vi "LTA-HS-testing2.vi"() -> ()   [LabVIEW 2013]
uses:
  <vilib>/Utility/error.llb/DialogType.ctl
panel:
  out "Current position":dbl
  out "error IO 2":errorcluster
  out "Motion Time (s)":dbl
  in  "Position":dbl
  in  "error IO":errorcluster
  in  "VISA resource name":refnum<visa-resource-name>
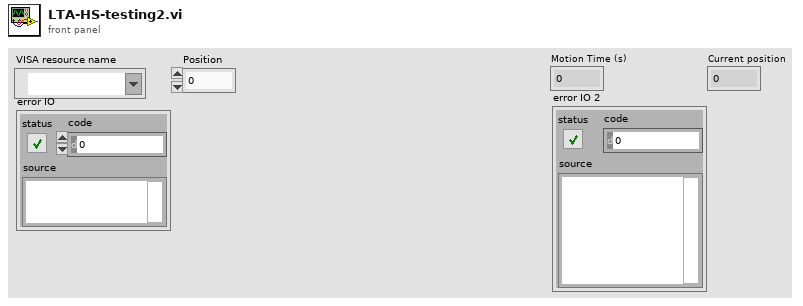
[diagram p1: front panel]
types:
  T1 = cluster{"VISA resource name":refnum<visa-resource-name>, string, i32, "error out":errorcluster}
  T2 = cluster{"VISA resource name":refnum<visa-resource-name>, "Device name":string, "Controller address":i32, "error":errorcluster}
  T3 = typedef "DialogType.ctl" = u16
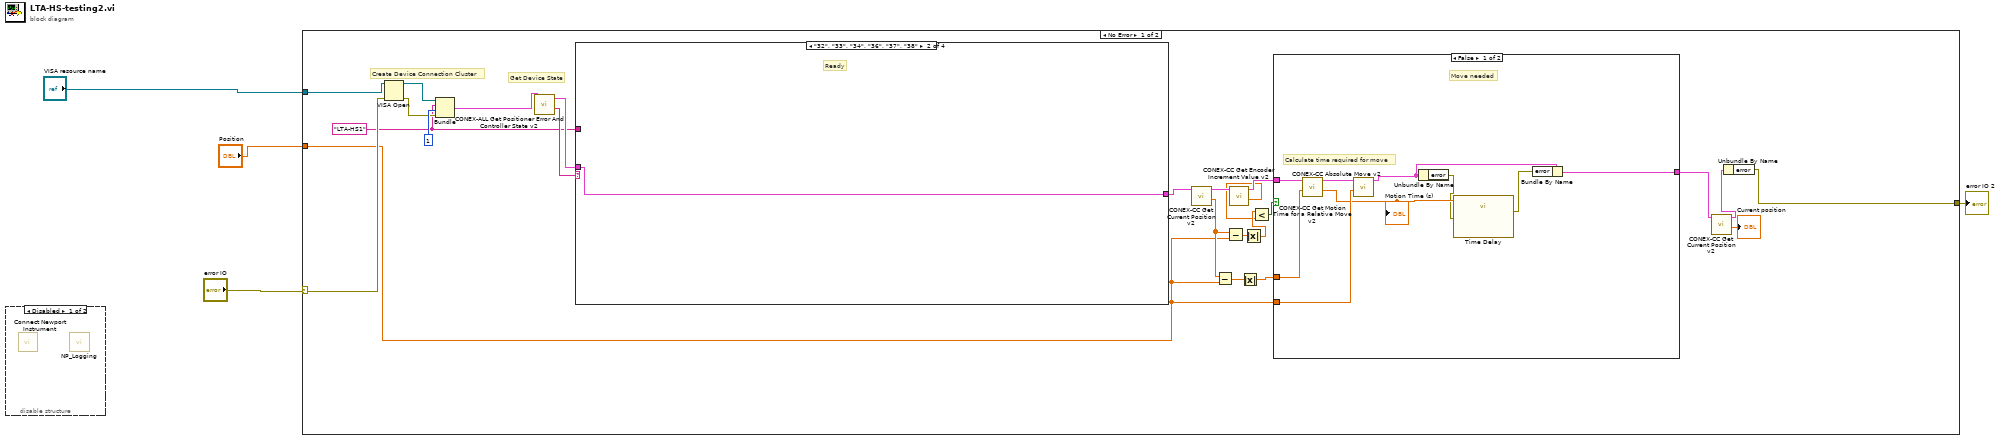
[diagram p0: block diagram]
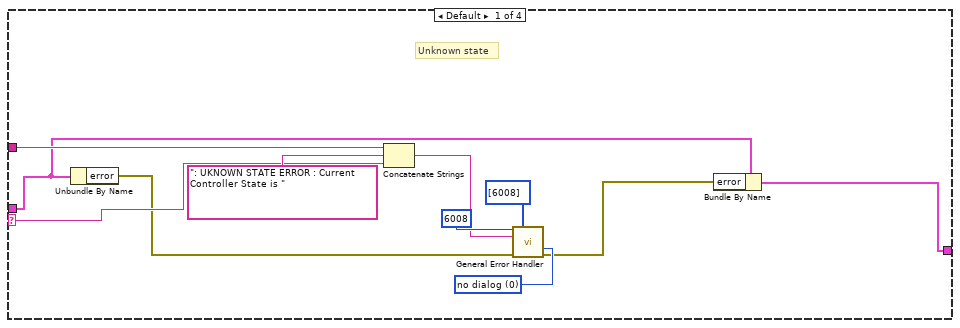
[diagram p4: hidden frame]
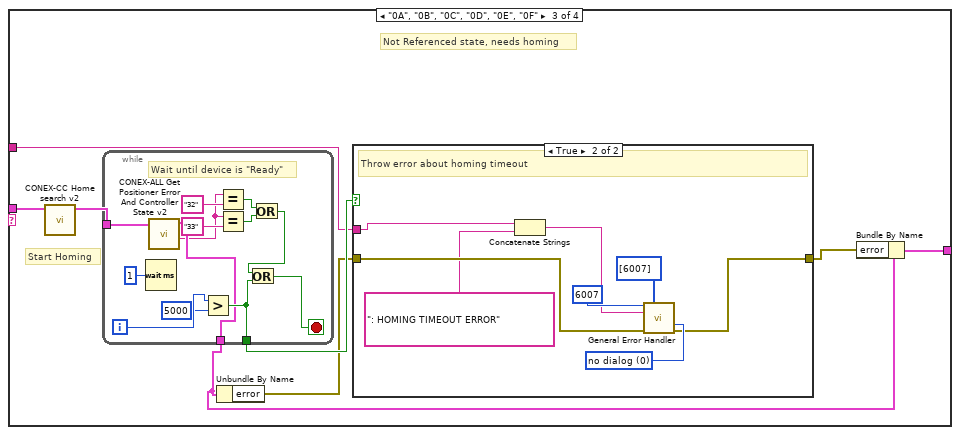
[diagram p5: hidden frame]
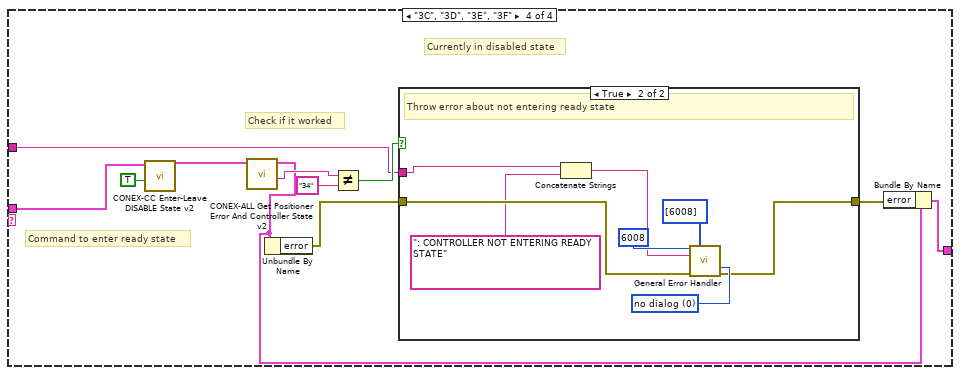
[diagram p7: hidden frame]
diagram:
  n1 = disable-structure shown="Disabled" {
    frame Disabled {
      n2 = call <userlib>:"Connect Newport Instrument.vi"() -> ()  [unwired: 7 in, 5 out]
      n3 = call <userlib>:"NP_Logging.vi"() -> ()  [unwired: 12 in, 4 out]
    }
    frame Enabled {
    }
  }
  n4 = case shown="No Error" "error IO" {
    selector: "error IO" -> [w25 w101]
    tunnel: [w18 w101] -> w1
    tunnel: "VISA resource name" -> [w16 _]
    tunnel: "Position" -> [w9 _]
    frame No Error {
      w17 = "LTA-HS1"
      # "Get Device State"
      # "Create Device Connection Cluster"
      n5 = VISA Open(error in (no error)=w25, VISA resource name=w16) -> (VISA resource name=w28:refnum<visa-resource-name>, error out=w26:errorcluster)  [unwired: 3 in]
      n6 = Bundle("VISA resource name"=w28, w17, 1, "error out"=w26) -> (w24:T1)  [unwired: 1 in]
      n7 = call <userlib>:"CONEX-ALL Get Positioner Error And Controller State v2.vi"("Connection Cluster in"=w24) -> ("Controller state"=w23:string, "Connection Cluster out"=w22:T2)  [unwired: 8 in, 1 out]
      n8 = case shown="\"32\", \"33\", \"34\", \"36\", \"37\", \"38\"" w23 {
        selector: w23 -> [w43 _ _ _]
        tunnel: w22 -> [w41 w50 w58 w91]
        tunnel: w17 -> [w44 _ w55 w85]
        tunnel: [w39 w50 w51 w81] -> w21
        frame Default {
          w49 = T3 0 items=["no dialog", "OK message", "continue or stop message", "OK message + warnings", "continue/stop + warnings"] ("type of dialog (OK msg:1)")
          # "Unknown state"
          n9 = Unbundle By Name(w41) -> ("error"=w42:errorcluster)
          n10 = Concatenate Strings(w44, ": UKNOWN STATE ERROR : Current Controller State is " ("format string"), w43) -> (w45:string)
          n11 = call <vilib>:"General Error Handler.vi"("[error code] (0)"=6008 ("error code (no error:0)"), "[user-defined codes]"=i32[] [6008], "[error source] (\" \")"=w45, "type of dialog (OK msg:1)"=w49, "error in (no error)"=w42) -> ("error out"=w40:errorcluster)  [unwired: 6 in, 4 out]
          n12 = Bundle By Name(cluster=w41, "error"=w40) -> (w39:T2)
        }
        frame "32", "33", "34", "36", "37", "38" {
          # "Ready"
        }
        frame "0A", "0B", "0C", "0D", "0E", "0F" {
          # "Start Homing"
          # "Not Referenced state, needs homing"
          n13 = call <userlib>:"CONEX-CC Home search v2.vi"("Connection Cluster in"=w58) -> ("Connection Cluster out"=w57:T2)  [unwired: 8 in]
          n14 = while {
            tunnel: w57 -> [w80]
            tunnel: [w70] -> w56
            tunnel: [w69] -> w53
            i -> [w72]
            stop <- w74 stop-if-true
            # "Wait until device is \"Ready\""
            n15 = Wait (ms)(milliseconds to wait=u32 1) -> ()  [unwired: 1 out]
            n16 = call <userlib>:"CONEX-ALL Get Positioner Error And Controller State v2.vi"("Connection Cluster in"=w80) -> ("Controller state"=w68:string, "Connection Cluster out"=w69:T2)  [unwired: 8 in, 1 out]
            n17 = Greater?(x=w72, y=5000) -> (0:w70:bool)
            n18 = Equal?(x=w68, y="32") -> (x = y?=w76:bool)
            n19 = Equal?(x=w68, y="33") -> (x = y?=w77:bool)
            n20 = Or(x=w76, y=w77) -> (x .or. y?=w75:bool)
            n21 = Or(x=w75, y=w70) -> (x .or. y?=w74:bool)
          }
          n22 = Unbundle By Name(w53) -> ("error"=w54:errorcluster)
          n23 = case shown="True" w56 {
            tunnel: w54 -> [w59 w66]
            tunnel: w55 -> [_ w62]
            tunnel: [w59 w64] -> w52
            frame False {
            }
            frame True {
              w67 = T3 0 items=["no dialog", "OK message", "continue or stop message", "OK message + warnings", "continue/stop + warnings"] ("type of dialog (OK msg:1)")
              # "Throw error about homing timeout"
              n24 = Concatenate Strings(w62, ": HOMING TIMEOUT ERROR" ("format string")) -> (w60:string)
              n25 = call <vilib>:"General Error Handler.vi"("[error code] (0)"=6007 ("error code (no error:0)"), "[user-defined codes]"=i32[] [6007], "[error source] (\" \")"=w60, "type of dialog (OK msg:1)"=w67, "error in (no error)"=w66) -> ("error out"=w64:errorcluster)  [unwired: 6 in, 4 out]
            }
          }
          n26 = Bundle By Name(cluster=w53, "error"=w52) -> (w51:T2)
        }
        frame "3C", "3D", "3E", "3F" {
          # "Check if it worked"
          # "Command to enter ready state"
          # "Currently in disabled state"
          n27 = call <userlib>:"CONEX-CC Enter-Leave DISABLE State v2.vi"("Ready? (false=DISABLE true=READY)"=TRUE, "Connection Cluster in"=w91) -> ("Connection Cluster out"=w89:T2)  [unwired: 7 in]
          n28 = call <userlib>:"CONEX-ALL Get Positioner Error And Controller State v2.vi"("Connection Cluster in"=w89) -> ("Controller state"=w87:string, "Connection Cluster out"=w83:T2)  [unwired: 8 in, 1 out]
          n29 = Unbundle By Name(w83) -> ("error"=w84:errorcluster)
          n30 = Not Equal?(x=w87, y="34") -> (x != y?=w86:bool)
          n31 = case shown="True" w86 {
            tunnel: w84 -> [w92 w99]
            tunnel: w85 -> [_ w95]
            tunnel: [w92 w97] -> w82
            frame False {
            }
            frame True {
              w100 = T3 0 items=["no dialog", "OK message", "continue or stop message", "OK message + warnings", "continue/stop + warnings"] ("type of dialog (OK msg:1)")
              # "Throw error about not entering ready state"
              n32 = Concatenate Strings(w95, ": CONTROLLER NOT ENTERING READY STATE" ("format string")) -> (w93:string)
              n33 = call <vilib>:"General Error Handler.vi"("[error code] (0)"=6008 ("error code (no error:0)"), "[user-defined codes]"=i32[] [6008], "[error source] (\" \")"=w93, "type of dialog (OK msg:1)"=w100, "error in (no error)"=w99) -> ("error out"=w97:errorcluster)  [unwired: 6 in, 4 out]
            }
          }
          n34 = Bundle By Name(cluster=w83, "error"=w82) -> (w81:T2)
        }
      }
      n35 = call <userlib>:"CONEX-CC Get Current Position v2.vi"("Connection Cluster in"=w21) -> ("Current position"=w10:dbl, "Connection Cluster out"=w12:T2)  [unwired: 8 in, 1 out]
      n36 = Subtract(x=w10, y=w9) -> (x-y=w20:dbl)
      n37 = Subtract(x=w10, y=w9) -> (x-y=w8:dbl)
      n38 = call <userlib>:"CONEX-CC Get Encoder Increment Value v2.vi"("Connection Cluster in"=w12) -> ("Encoder Increment Value"=w6:dbl, "Connection Cluster out"=w11:T2)  [unwired: 8 in, 1 out]
      n39 = Absolute Value(x=w20) -> (abs(x)=w19:dbl)
      n40 = Absolute Value(x=w8) -> (abs(x)=w7:dbl)
      n41 = Less?(x=w7, y=w6) -> (x < y?=w5:bool)
      n42 = case shown="False" w5 {
        tunnel: w19 -> [w37 _]
        tunnel: w9 -> [w35 _]
        tunnel: [w30 w38] -> w14
        tunnel: w11 -> [w29 w38]
        frame False {
          # "Calculate time required for move"
          # "Move needed"
          n43 = call <userlib>:"CONEX-CC Get Motion Time for a Relative Move v2.vi"("Displacement"=w37, "Connection Cluster in"=w29) -> ("Motion Time (s)"=w34:dbl, "Connection Cluster out"=w36:T2)  [unwired: 7 in, 1 out]
          "Motion Time (s)" <- w34
          n44 = call <userlib>:"CONEX-CC Absolute Move v2.vi"("Target position"=w35, "Connection Cluster in"=w36) -> ("Connection Cluster out"=w32:T2)  [unwired: 7 in]
          n45 = Unbundle By Name(w32) -> ("error"=w33:errorcluster)
          n46 = call "Time Delay"("error in (no error)"=w33, "Delay Time (s)"=w34) -> ("error out"=w31:errorcluster)  [unwired: 9 in]
          n47 = Bundle By Name(cluster=w32, "error"=w31) -> (w30:T2)
        }
        frame True {
          # "Current position = Target Position"
        }
      }
      n48 = call <userlib>:"CONEX-CC Get Current Position v2.vi"("Connection Cluster in"=w14) -> ("Current position"=→"Current position":dbl, "Connection Cluster out"=w13:T2)  [unwired: 8 in, 1 out]
      n49 = Unbundle By Name(w13) -> ("error"=w18:errorcluster)
    }
    frame Error {
    }
  }
  "error IO 2" <- w1
